vi "Count samples.vi"(8 "input valid":bool=TRUE, 10 "Samples to count":fxp<+,16,16>, 11 "Reset":bool) -> (0 "output valid":bool, 2 "counting":bool)   [LabVIEW 2013]
uses:
  <vilib>/rvi/FXPMathLib/FxpSub/XNode/nifxpmath_Sub.xnode
  <vilib>/rvi/FXPMathLib/sim/FxpSim.dll
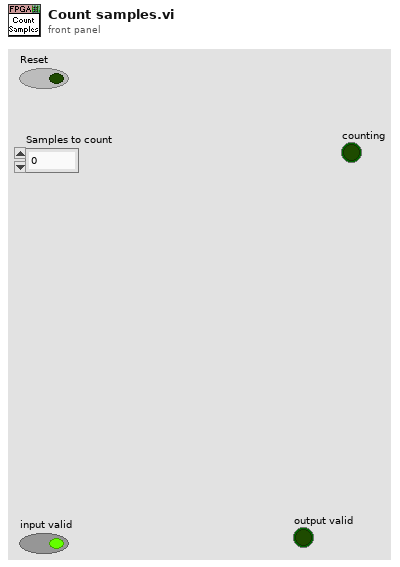
[diagram p1: front panel]
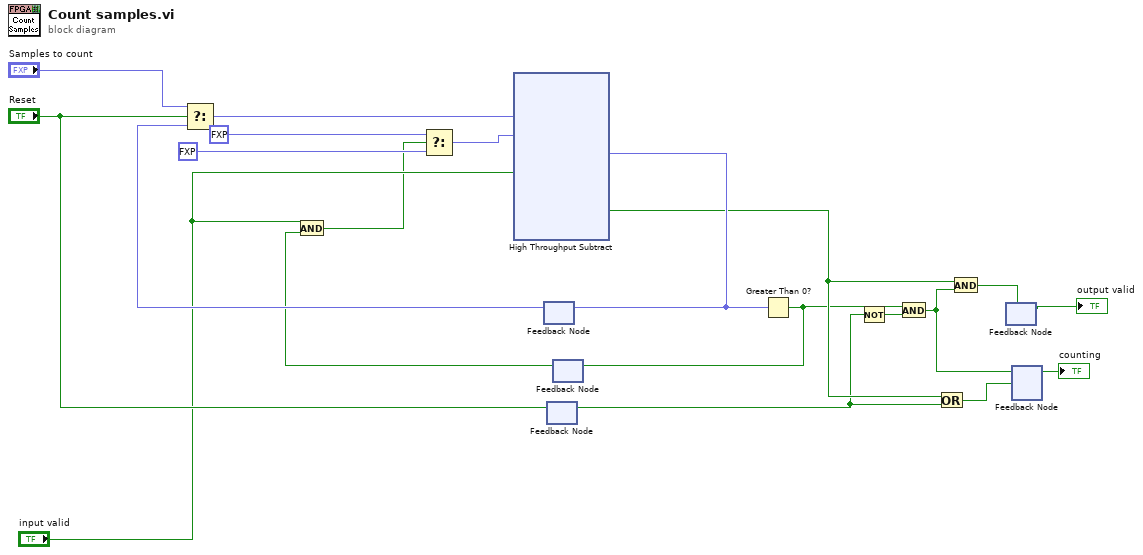
[diagram p0: block diagram]
diagram:
  n1 = feedback #1() -> (w16:fxp<+,16,16>)  [unwired: 1 in]
  n2 = Select(t="Samples to count", s="Reset", f=w16) -> (s? t:f=w19:fxp<+,16,16>)
  n3 = feedback #2() -> (w4:bool)  [unwired: 1 in]
  n4 = feedback-in #2("Reset") -> ()
  n5 = feedback #3() -> (w6:bool)  [unwired: 1 in]
  n6 = And(x="input valid", y=w6) -> (x .and. y?=w5:bool)
  n7 = Select(t=fxp<+,16,16> 1.0 ("y"), s=w5, f=fxp<+,16,16> 0.0 ("y")) -> (s? t:f=w14:fxp<+,16,16>)
  n8 = xnode "High Throughput Subtract"("x"=w19, "y"=w14, "input valid"="input valid") -> ("x-y"=w15:fxp<+,16,16>, "output valid"=w9:bool)  [unwired: 1 in, 1 out]
  n9 = feedback-in #1(w15) -> ()
  n10 = Greater Than 0?(x=w15) -> (x > 0?=w2:bool)
  n11 = feedback-in #3(w2) -> ()
  n12 = Not(x=w4) -> (.not. x?=w3:bool)
  n13 = And(x=w2, y=w3) -> (x .and. y?=w1:bool)
  n14 = Or(x=w9, y=w4) -> (x .or. y?=w8:bool)
  n15 = And(x=w9, y=w1) -> (x .and. y?=w12:bool)
  n16 = feedback-in #4(w12) -> ()
  n17 = feedback #4() -> (→"output valid":bool)  [unwired: 1 in]
  n18 = feedback-in #5(w1, w8) -> ()
  n19 = feedback #5() -> (→"counting":bool)  [unwired: 1 in]
